vi "sub_gen_pilot_carriers.vi"(9 "message carrier":i32=120, 11 "FFT size":i32=256) -> (0 "RX pilot carriers":cdb[](array[numeric]), 3 "TX pilot carriers":cdb[](array[numeric]))   [LabVIEW 2014]
uses:
  <vilib>/addons/Modulation/Digital/General/MT Generate PSK System Parameters(M).vi
  <vilib>/addons/Modulation/niDMT.lvlib
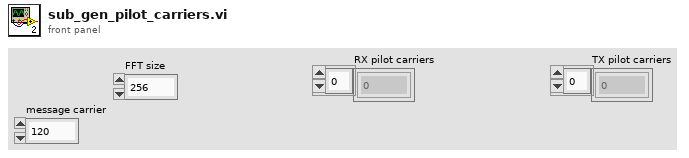
[diagram p1: front panel]
types:
  T1 = cluster{"samples per symbol (16)":i32, "symbol map":cdb[], "differential PSK":enum16{"disable", "enable"}, "PSK type":u16}
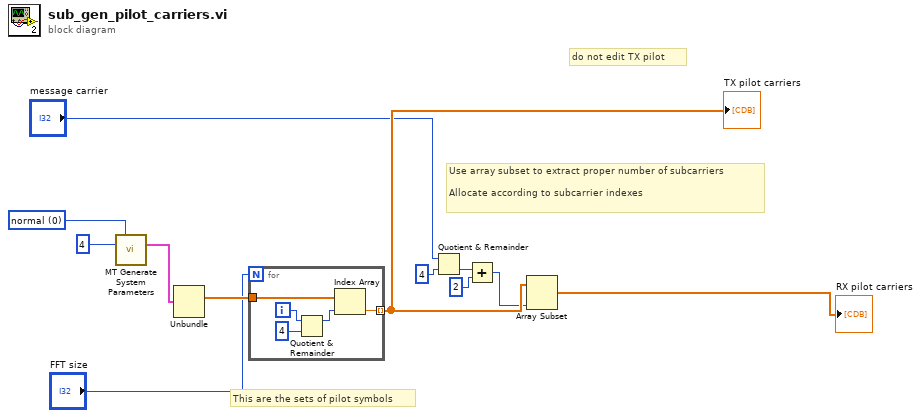
[diagram p0: block diagram]
diagram:
  w12 = u16 0 items=["normal", "shifted", "offset"] ("PSK type")
  # "Use array subset to extract proper number of subcarriers\n\nAllocate according to subcarrier indexes"
  # "This are the sets of pilot symbols"
  # "do not edit TX pilot"
  n1 = call-poly <vilib>:"MT Generate System Parameters.vi"("PSK type"=w12, "M-PSK (4)"=4) -> ("PSK system parameters"=w10:T1)  [unwired: 11 in, 2 out]
  n2 = Unbundle(w10) -> ("symbol map"=w9:cdb[])  [unwired: 3 out]
  n3 = for {
    N: "FFT size" -> [_]
    tunnel: w9 -> [w15]
    tunnel: [w13] -> w7 mode=indexing
    i -> [w17]
    n4 = Quotient & Remainder(x=w17, y=4) -> (x-y*floor(x/y)=w14:i32)  [unwired: 1 out]
    n5 = Index Array(array=w15, index=w14) -> (element=w13:cdb)
  }
  "TX pilot carriers" <- w7
  n6 = Quotient & Remainder(x="message carrier", y=4) -> (floor(x/y)=w5:i32)  [unwired: 1 out]
  n7 = Add(x=w5, y=2) -> (x+y=w2:i32)
  n8 = Array Subset(array=w7, length=w2) -> (→"RX pilot carriers":cdb[])  [unwired: 1 in]
